vi "Load Package Config.vi"(0 "Path":path, 11 "Error In":errorcluster) -> (3 "Path Out":path[](array[path]), 4 "Package ID":string, 6 "Purpose":string, 8 "Package Revision":string, 10 "MD5 Chk sum":string[](array[string]), 15 "Error Out":errorcluster)   [LabVIEW 2010]
uses:
  <vilib>/Utility/config.llb/Read Key (String).vi
  <vilib>/Utility/config.llb/NI_LVConfig.lvlib
panel:
  out "Array":string[](array[string])
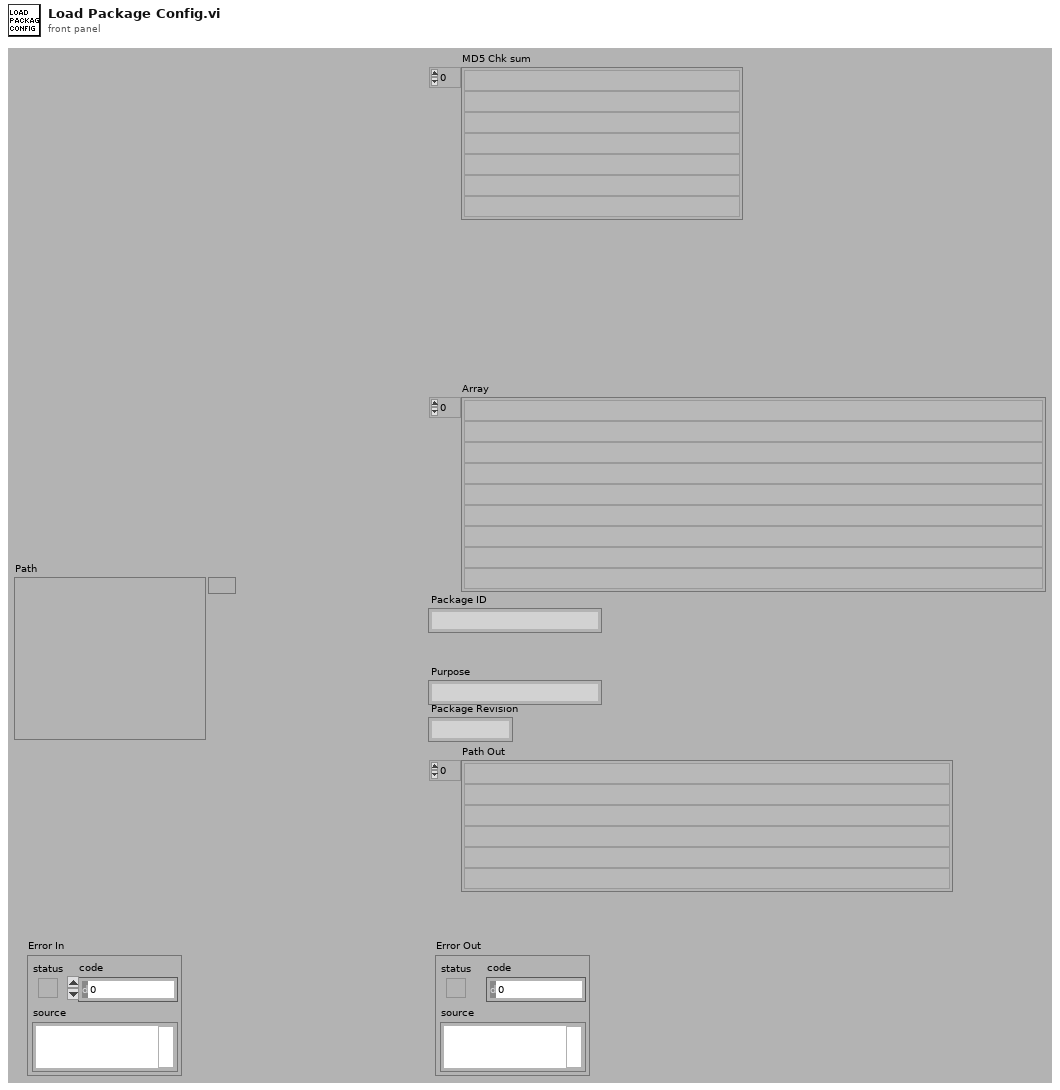
[diagram p1: front panel]
types:
  T1 = typedef "NI_LVConfig.lvlib/Config Data RefNum.ctl" = refnum<k1>
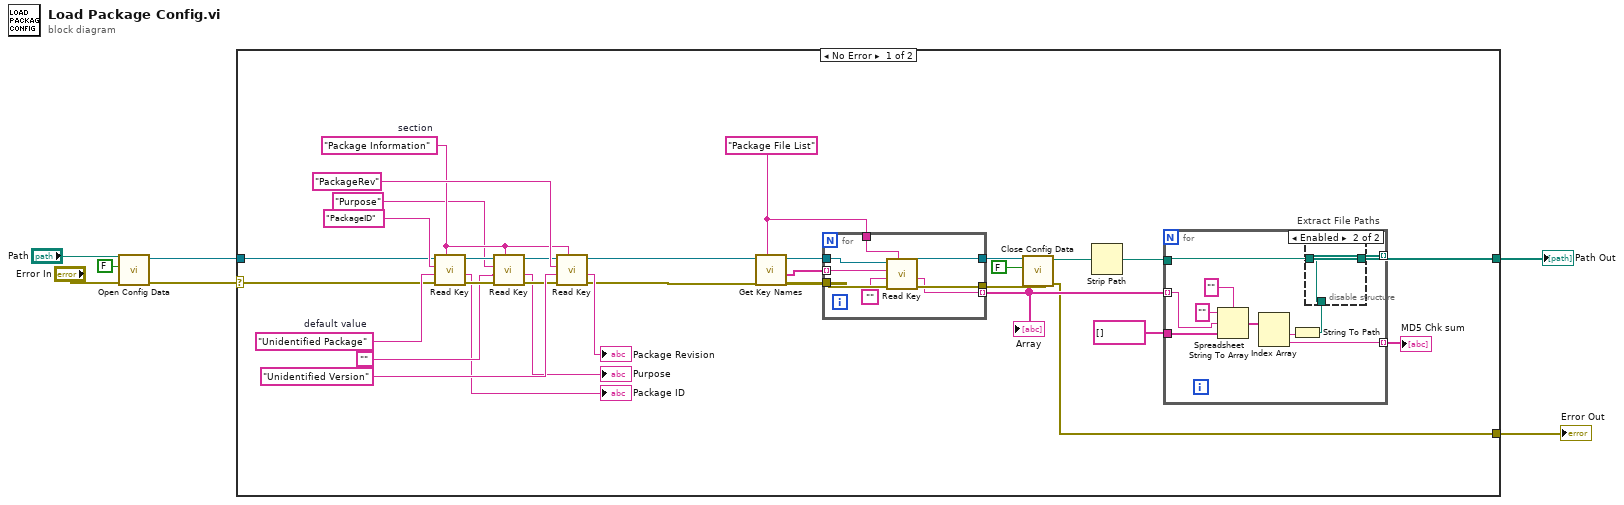
[diagram p0: block diagram]
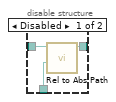
[diagram p2: hidden frame]
diagram:
  n1 = call <vilib>:"Open Config Data.vi"("error in (no error)"="Error In", "create file if necessary (T)"=FALSE, "configuration file path"="Path") -> ("error out"=w1:errorcluster, "refnum"=w7:T1)  [unwired: 6 in, 1 out]
  n2 = case shown="No Error" w1 {
    selector: w1 -> [w9 _]
    tunnel: w7 -> [w35 _]
    tunnel: [w22 _] -> w4
    tunnel: [w10 _] -> w2
    frame No Error {
      w38 = "Unidentified Package"  # default value
      w30 = "Package Information"  # section
      w18 = "Package File List" ("section")
      n3 = call-poly <vilib>:"Read Key.vi"("section"=w30, "error in (no error)"=w9, "default value"=w38, "key"="PackageID", "refnum"=w35) -> ("error out"=w34:errorcluster, "value"=→"Package ID":string, "refnum out"=w33:T1)  [unwired: 3 in, 1 out]
      n4 = call-poly <vilib>:"Read Key.vi"("section"=w30, "error in (no error)"=w34, "default value"="", "key"="Purpose", "refnum"=w33) -> ("error out"=w31:errorcluster, "value"=→"Purpose":string, "refnum out"=w32:T1)  [unwired: 3 in, 1 out]
      n5 = call-poly <vilib>:"Read Key.vi"("section"=w30, "error in (no error)"=w31, "default value"="Unidentified Version", "key"="PackageRev", "refnum"=w32) -> ("error out"=w20:errorcluster, "value"=→"Package Revision":string, "refnum out"=w21:T1)  [unwired: 3 in, 1 out]
      n6 = call <vilib>:"Get Key Names.vi"("section"=w18, "error in (no error)"=w20, "refnum"=w21) -> ("error out"=w17:errorcluster, "key names"=w19:string[], "refnum out"=w16:T1)  [unwired: 5 in, 1 out]
      n7 = for {
        tunnel: w19 -> [w47] mode=indexing
        tunnel: w18 -> [w46]
        tunnel: w17 -> [w45]
        tunnel: [w44] -> w15
        tunnel: w16 -> [w43]
        tunnel: [w42] -> w14
        tunnel: [w40] -> w13 mode=indexing
        n8 = call-poly <vilib>:"Read Key.vi"("section"=w46, "error in (no error)"=w45, "default value"="", "key"=w47, "refnum"=w43) -> ("error out"=w44:errorcluster, "value"=w40:string, "refnum out"=w42:T1)  [unwired: 3 in, 1 out]
      }
      "Array" <- w13
      n9 = call <vilib>:"Close Config Data.vi"("error in (no error)"=w15, "write file if changed (T)"=FALSE, "refnum"=w14) -> ("error out"=w10:errorcluster, "file path"=w26:path)  [unwired: 7 in]
      n10 = Strip Path(path=w26) -> (stripped path=w12:path)  [unwired: 1 out]
      n11 = for "Extract File Paths" {
        tunnel: w13 -> [w49] mode=indexing
        tunnel: [w56] -> w22 mode=indexing
        tunnel: w12 -> [w55]
        tunnel: string[] [] -> [w54]
        tunnel: [w48] -> w8 mode=indexing
        n12 = Spreadsheet String To Array(delimiter (Tab)="" ("format string"), format string="", spreadsheet string=w49, array type (2D Dbl)=w54) -> (array=w52:string[])
        n13 = Index Array(array=w52) -> (element #1=w51:string, element #2=w48:string)  [unwired: 2 in]
        n14 = String To Path(string=w51) -> (path=w57:path)
        n15 = disable-structure shown="Enabled" {
          disable-tunnel: w57 -> [w60 w61]
          disable-tunnel: [w59 w61] -> w56
          disable-tunnel: w55 -> [w58 _]
          frame Disabled {
            n16 = call "Rel to Abs Path.vi"("Rel File Path"=w60, "Base Path"=w58) -> ("Path Out"=w59:path)  [unwired: 8 in, 1 out]
          }
          frame Enabled {
          }
        }
      }
      "MD5 Chk sum" <- w8
    }
    frame Error {
    }
  }
  "Path Out" <- w4
  "Error Out" <- w2
